vi "Random Seas (math only).vi"() -> ()   [LabVIEW 2012]
uses:
  Instance           2 19Saved   Random Seas .vi
  Instance           1 19Saved   Random Seas .vi
panel:
  out "File Name Out":path
  out "Wavestaff Signal":dbl[](graph)
  in  "Measure Waves":bool
  in  "Input Settings":bool
  in  "Geometric Settings":bool
  in  "Limit Settings":bool
  in  "Output Settings":bool
  out "Output Sig. Wave Height":dbl format="%.4f"
  out "Buffer Completed":dbl format="%.1f"
  out "Time Series Data":dbl[](array[numeric]) format="%.2f"
  out "Output Signal":dbl[](graph)
  in  "Set spectal parameters":bool
  in  "Run":bool
  in  "Power":bool
  out "Significant Wave Period":dbl format="%.4f"
  out "Significant Wave Height":dbl format="%.4f"
  in  "Select spectrum":u16(ring) items=["Bretschnieder", "JONSWAP", "NH Extreme", "NH Typical", "Pierson Moskowitz"]
  out "Spectra":cluster{"Numeric":dbl, "Numeric":dbl}[](graph)
  out "Time Series":cluster{"Numeric":dbl, "Numeric":sgl}[](graph)
  # "Random Sea Generator"
  # "m"
  # "s"
  # "Time (min:sec)"
  # "%"
  # "m"
  # "Time (min:sec)"
  # "Frequency (Hz)"
  # "Advanced"
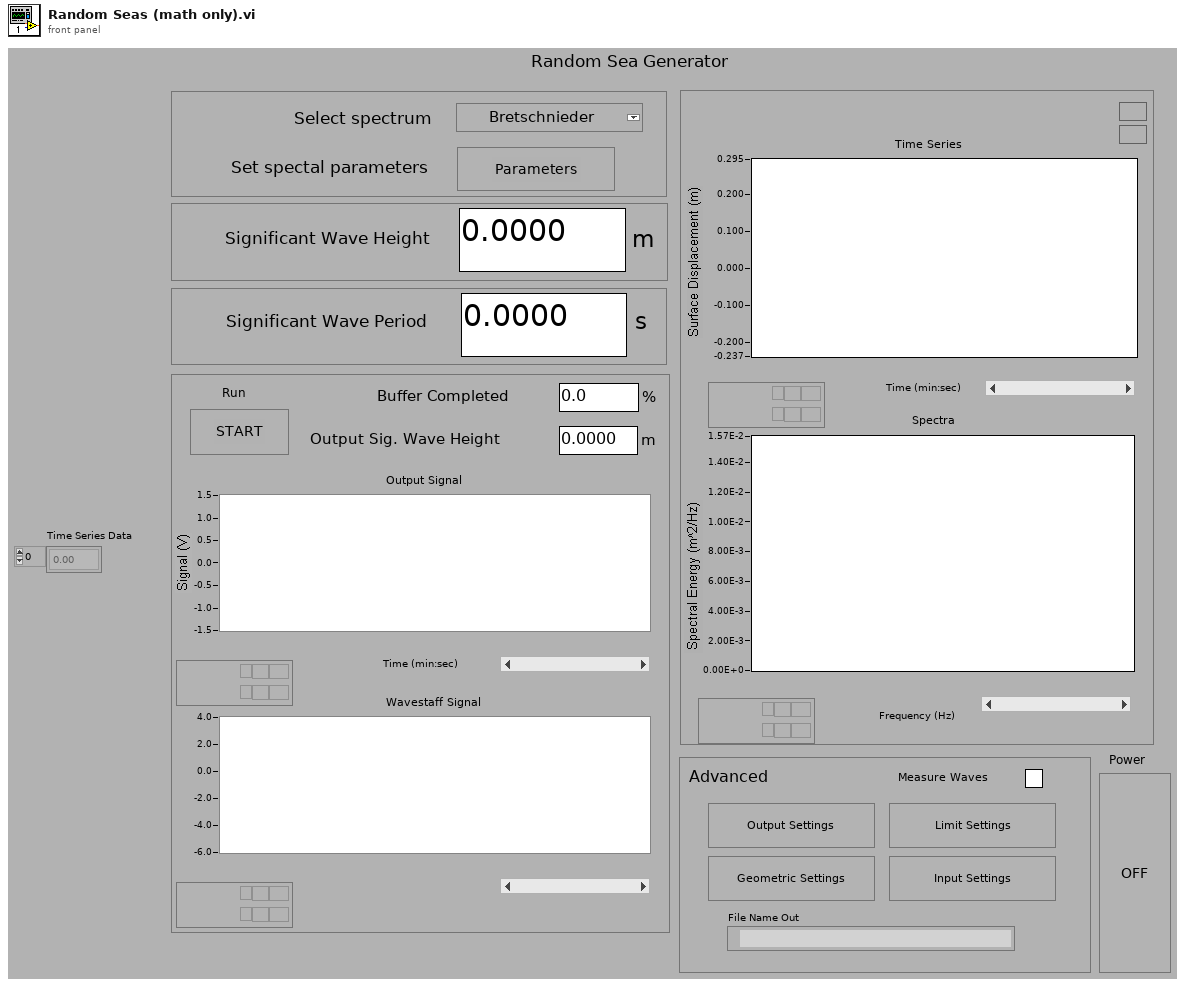
[diagram p1: front panel]
types:
  T1 = cluster{"Input Device":i32, "Input Channel":string, "Input Offset":dbl, "Input Calibration":dbl}
  T2 = cluster{"Device":i16, "Channel":string, "Sampling Rate":i32, "Ramp Time":dbl, "Buffer Length":u16, "Buffer Size":i32, "Sub Buffer Length":i16, "Sub Buffer Size":i16}
  T3 = cluster{"Stroke Calibration":dbl, "Water Depth":dbl, "Paddle Height":dbl}
  T4 = cluster{"Min Wave Period":dbl, "Max Wave Period":dbl, "Cutoff Frequency":dbl, "Max 1/2 Piston Stroke":dbl, "Max H/L":dbl, "Max H/d":dbl}
  T5 = cluster{"Bretschneider":cluster{"Sig Wave Height":dbl, "Sig Wave Period":dbl, "Scale Ratio":dbl}, "JONSWAP":cluster{"Sig Wave Height":dbl, "Sig Wave Period":dbl, "Gamma":dbl, "Sigma A":dbl, "Sigma B":dbl, "Scale Ratio":dbl}, "NH Extreme":cluster{"Sig Wave Height":dbl, "Sig Wave Period":dbl, "Gamma":dbl, "Sigma A":dbl, "Sigma B":dbl, "P":dbl, "Scale Ratio":dbl}, "NH Typical":cluster{"Sig Wave Height":dbl, "Sig Wave Period 1":dbl, "Sig Wave Period 2":dbl, "Gamma 1":dbl, "Gamma 2":dbl, "P":dbl, "Scale Ratio":dbl}, "PM":cluster{"Wind speed":dbl, "Scale Ratio":dbl}}
  T6 = cluster{"Element Data":dbl, "Element Data":dbl}[]
  T7 = cluster{"Sig Wave Height":dbl, "Sig Wave Period":dbl, "Scale Ratio":dbl}
  T8 = cluster{"Sig Wave Height":dbl, "Sig Wave Period":dbl, "Gamma":dbl, "Sigma A":dbl, "Sigma B":dbl, "Scale Ratio":dbl}
  T9 = cluster{"Sig Wave Height":dbl, "Sig Wave Period":dbl, "Gamma":dbl, "Sigma A":dbl, "Sigma B":dbl, "P":dbl, "Scale Ratio":dbl}
  T10 = cluster{"Sig Wave Height":dbl, "Sig Wave Period":dbl, "Sig Wave Period 2":dbl, "Gamma 1":dbl, "Gamma 2":dbl, "P":dbl, "Scale Ratio":dbl}
  T11 = cluster{"Device":i16, "Channel":string, "Sampling Rate":i32, "Stroke Calibration":dbl, "Buffer Length":u16, "Buffer Size":i32, "Sub Buffer Length":i16, "Sub Buffer Size":i16}
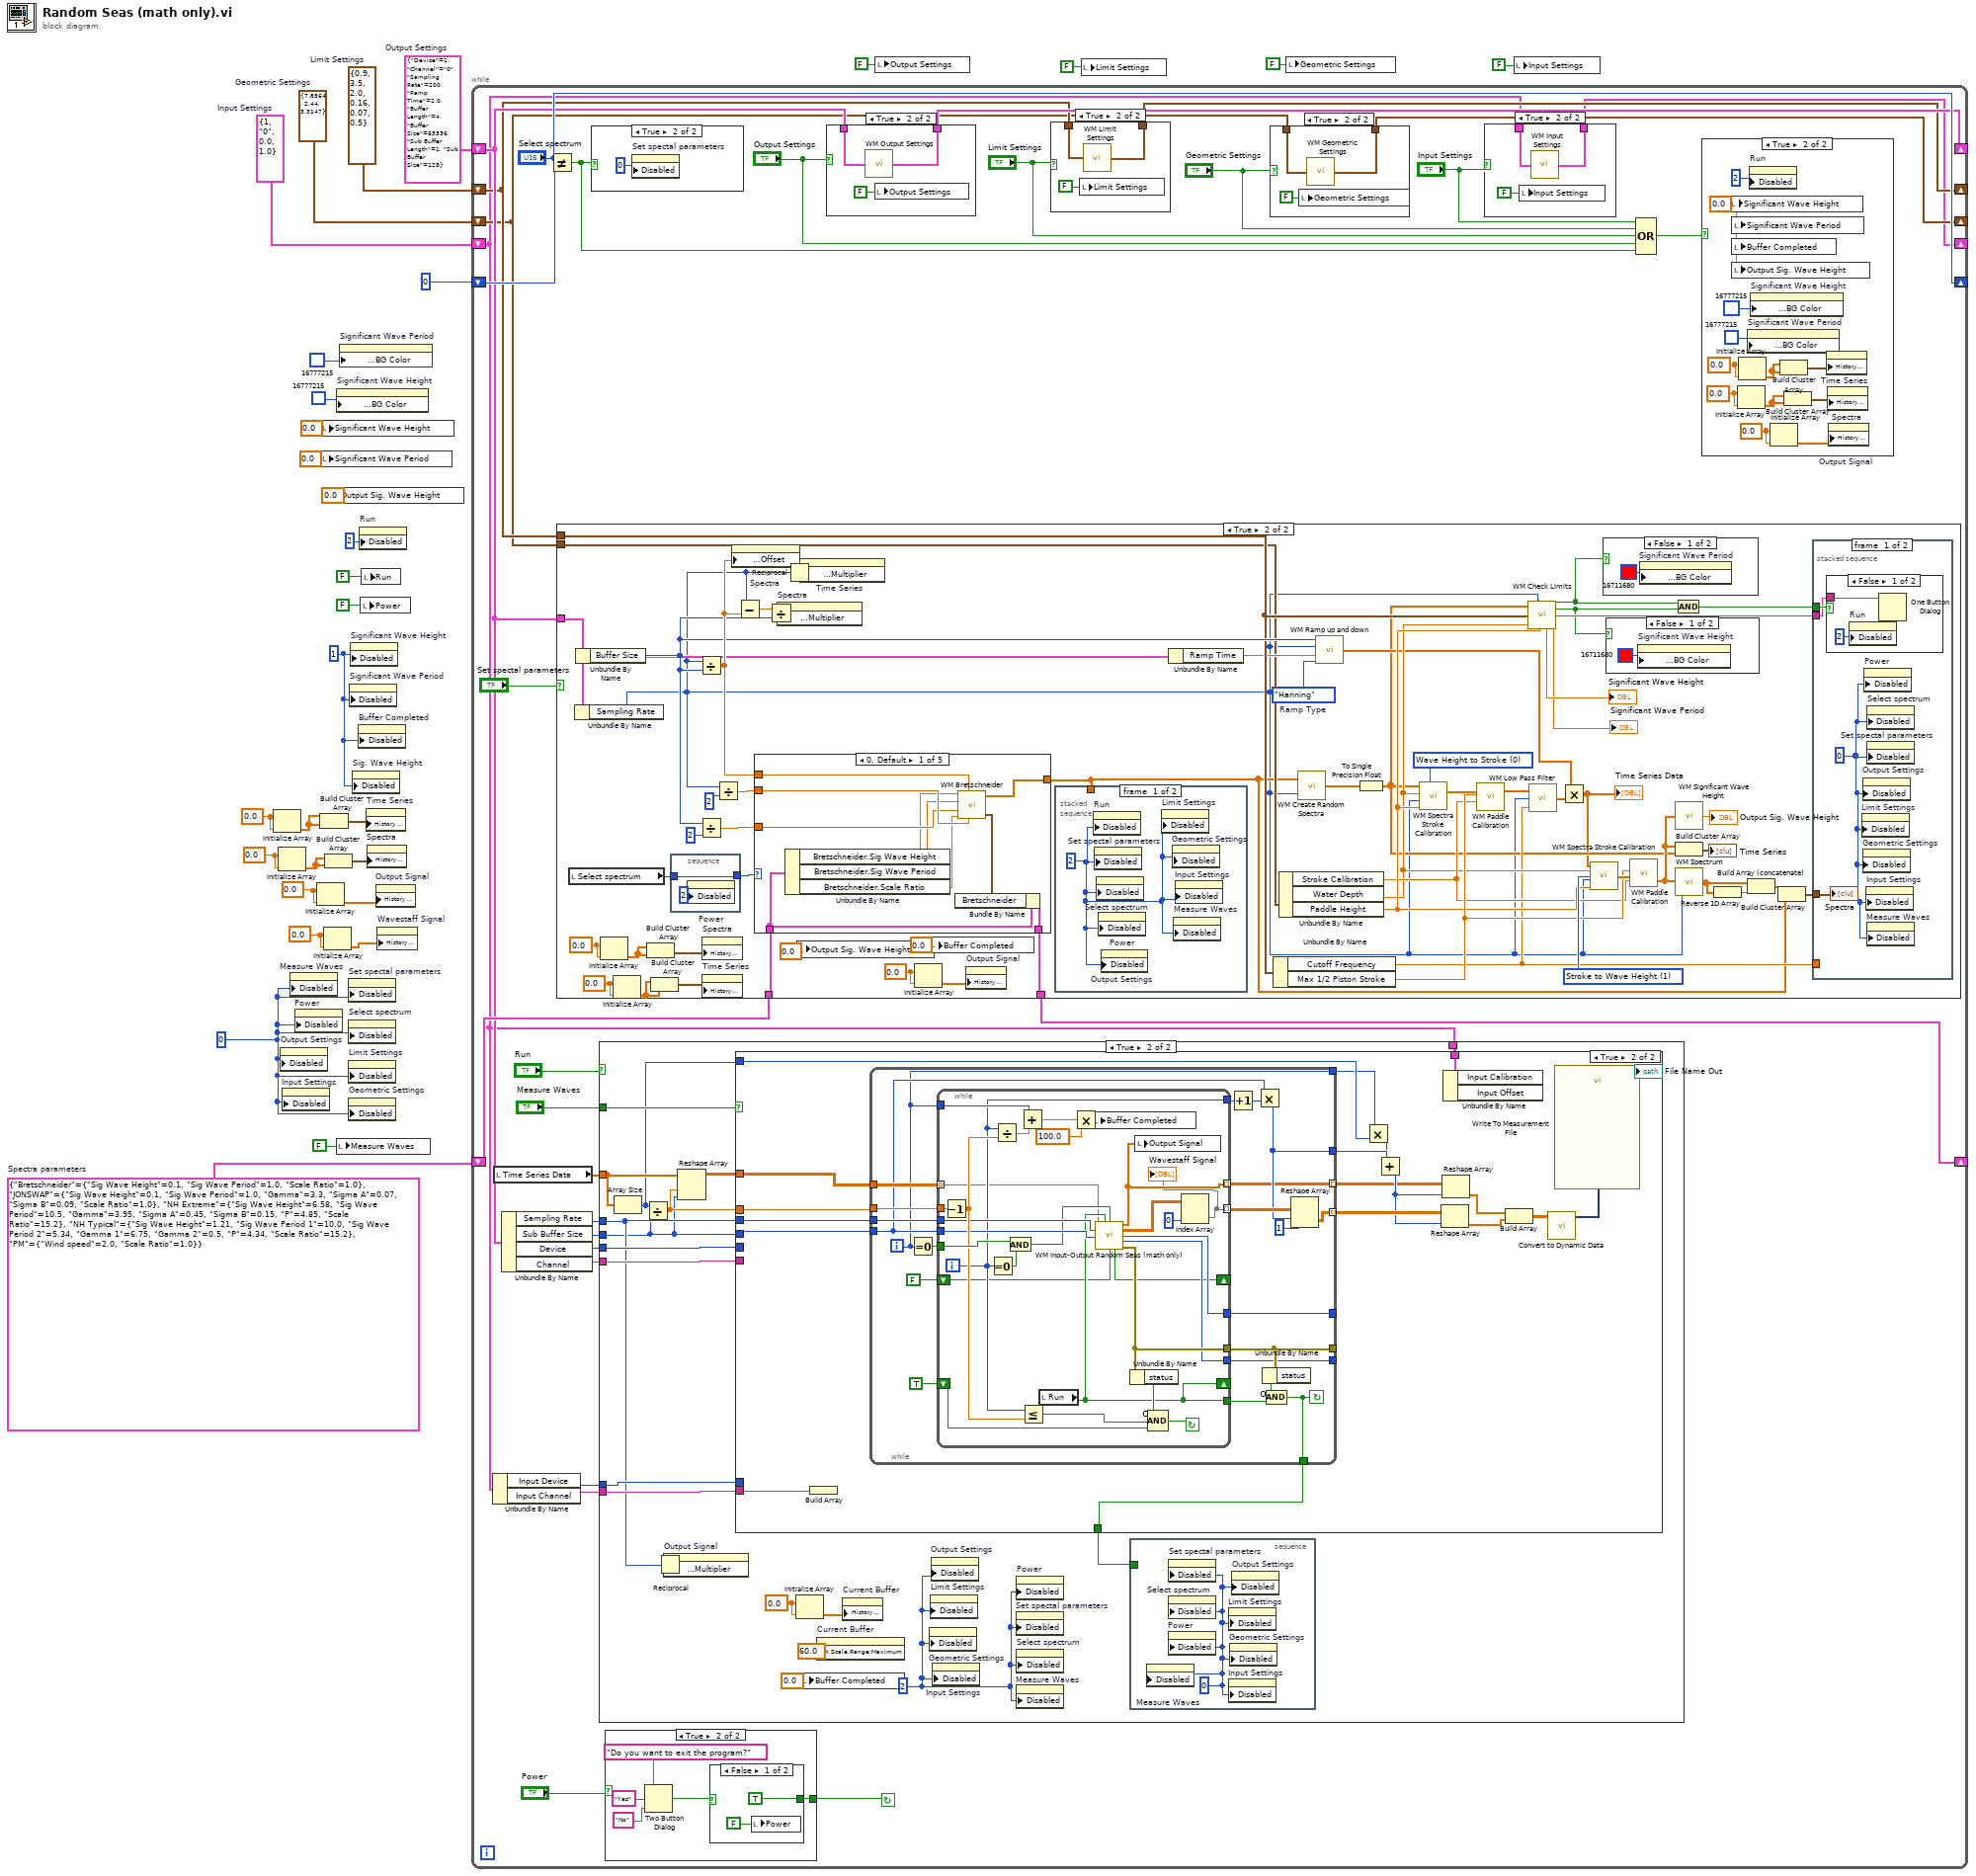
[diagram p0: block diagram]
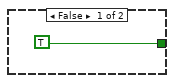
[diagram p7: hidden frame]
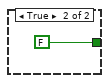
[diagram p8: hidden frame]
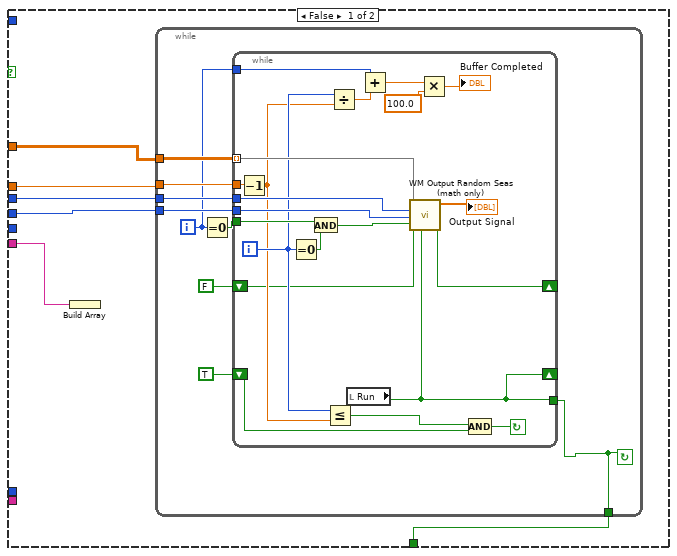
[diagram p11: hidden frame]
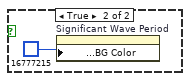
[diagram p13: hidden frame]
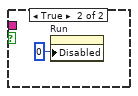
[diagram p15: hidden frame]
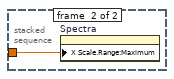
[diagram p16: hidden frame]
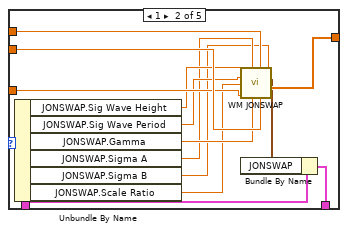
[diagram p17: hidden frame]
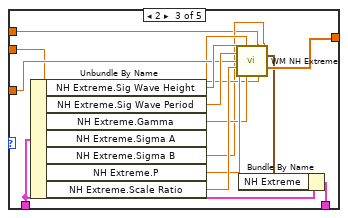
[diagram p18: hidden frame]
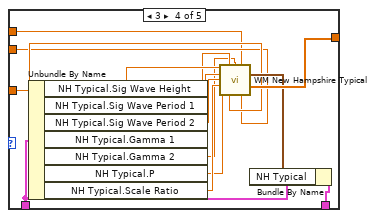
[diagram p19: hidden frame]
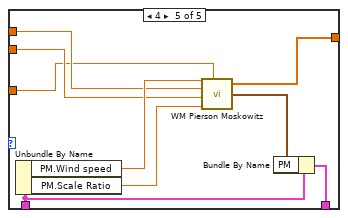
[diagram p20: hidden frame]
diagram:
  w2 = 0.0 ("Element Data")
  w5 = T1 {"Input Device"=1, "Input Channel"="0", "Input Offset"=0.0, "Input Calibration"=1.0}  # Input Settings
  w8 = T2 {"Device"=1, "Channel"="0", "Sampling Rate"=200, "Ramp Time"=2.0, "Buffer Length"=4, "Buffer Size"=65536, "Sub Buffer Length"=1, "Sub Buffer Size"=128}  # Output Settings
  w10 = T3 {"Stroke Calibration"=7.8564, "Water Depth"=2.44, "Paddle Height"=3.3147}  # Geometric Settings
  w11 = T4 {"Min Wave Period"=0.9, "Max Wave Period"=3.5, "Cutoff Frequency"=2.0, "Max 1/2 Piston Stroke"=0.16, "Max H/L"=0.07, "Max H/d"=0.5}  # Limit Settings
  w16 = 0.0 ("Element Data")
  w3 = u8 0 ("Write Attribute")
  w27 = 0.0 ("Element Data")
  w28 = 0.0 ("Element Data")
  w25 = T5 {"Bretschneider"={"Sig Wave Height"=0.1, "Sig Wave Period"=1.0, "Scale Ratio"=1.0}, "JONSWAP"={"Sig Wave Height"=0.1, "Sig Wave Period"=1.0, "Gamma"=3.3, "Sigma A"=0.07, "Sigma B"=0.09, "Scale Ratio"=1.0}, "NH Extreme"={"Sig Wave Height"=6.58, "Sig Wave Period"=10.5, "Gamma"=3.95, "Sigma A"=0.45, "Sigma B"=0.15, "P"=4.85, "Scale Ratio"=15.2}, "NH Typical"={"Sig Wave Height"=1.21, "Sig Wave Period 1"=10.0, "Sig Wave Period 2"=5.34, "Gamma 1"=6.75, "Gamma 2"=0.5, "P"=4.34, "Scale Ratio"=15.2}, "PM"={"Wind speed"=2.0, "Scale Ratio"=1.0}}  # Spectra parameters
  w9 = 1
  n1 = Initialize Array(w28, w28) -> (w18:dbl[])
  n2 = Initialize Array(w27, w27) -> (w26:dbl[])
  n3 = property on="Output Settings" class="Bool (strict)"("Disabled"=w3) -> ()  [unwired: 2 in, 2 out]
  n4 = property on="Input Settings" class="Bool (strict)"("Disabled"=w3) -> ()  [unwired: 2 in, 2 out]
  n5 = property on="Measure Waves" class="Bool (strict)"("Disabled"=w3) -> ()  [unwired: 2 in, 2 out]
  n6 = property on="Power" class="Bool (strict)"("Disabled"=w3) -> ()  [unwired: 2 in, 2 out]
  n7 = Initialize Array(w16, w16) -> (w15:dbl[])
  n8 = local write "Significant Wave Height"(0.0 ("Significant Wave Height")) -> ()
  n9 = local write "Significant Wave Period"(0.0 ("Significant Wave Period")) -> ()
  n10 = Build Cluster Array(w18, w18) -> (w17:T6)
  n11 = Initialize Array(w2, w2) -> (w1:dbl[])
  n12 = Build Cluster Array(w26, w26) -> (w19:T6)
  n13 = local write "Output Sig. Wave Height"(0.0 ("Sig. Wave Height")) -> ()
  n14 = property on="Significant Wave Height" class="DigNum (strict)"("Numeric Text.Text Colors:BG Color"=u32 16777215) -> ()  [unwired: 2 in, 2 out]
  n15 = local write "Measure Waves"(FALSE ("Measure Waves")) -> ()
  n16 = property on="Significant Wave Period" class="DigNum (strict)"("Numeric Text.Text Colors:BG Color"=u32 16777215) -> ()  [unwired: 2 in, 2 out]
  n17 = property on="Set spectal parameters" class="Bool"("Disabled"=w3) -> ()  [unwired: 2 in, 2 out]
  n18 = property on="Select spectrum" class="Ring (strict)"("Disabled"=w3) -> ()  [unwired: 2 in, 2 out]
  n19 = property on="Limit Settings" class="Bool (strict)"("Disabled"=w3) -> ()  [unwired: 2 in, 2 out]
  n20 = property on="Geometric Settings" class="Bool (strict)"("Disabled"=w3) -> ()  [unwired: 2 in, 2 out]
  n21 = property on="Significant Wave Period" class="DigNum (strict)"("Disabled"=w9) -> ()  [unwired: 2 in, 2 out]
  n22 = property on="Significant Wave Height" class="DigNum (strict)"("Disabled"=w9) -> ()  [unwired: 2 in, 2 out]
  n23 = property on="Sig. Wave Height" class="DigNum (strict)"("Disabled"=w9) -> ()  [unwired: 2 in, 2 out]
  n24 = property on="Buffer Completed" class="DigNum (strict)"("Disabled"=w9) -> ()  [unwired: 2 in, 2 out]
  n25 = property on="Run" class="Bool (strict)"("Disabled"=u8 2 ("Write Attribute")) -> ()  [unwired: 2 in, 2 out]
  n26 = local write "Power"(FALSE ("Power")) -> ()
  n27 = local write "Run"(FALSE ("Run")) -> ()
  n28 = property on="Time Series" class="WFChart (strict)"("History Data"=w17) -> ()  [unwired: 2 in, 2 out]
  n29 = property on="Spectra" class="WFChart (strict)"("History Data"=w19) -> ()  [unwired: 2 in, 2 out]
  n30 = property on="Output Signal" class="WFChart (strict)"("History Data"=w15) -> ()  [unwired: 2 in, 2 out]
  n31 = property on="Wavestaff Signal" class="WFChart (strict)"("History Data"=w1) -> ()  [unwired: 2 in, 2 out]
  n32 = while {
    shift-left: w5 -> [w32]
    shift-right: [w42] -> _
    shift-left: w10 -> [w43]
    shift-right: [w44] -> _
    shift-left: w11 -> [w45]
    shift-right: [w46] -> _
    shift-left: w8 -> [w51]
    shift-right: [w52] -> _
    shift-left: 0 -> [w55]
    shift-right: ["Select spectrum"] -> _
    shift-left: w25 -> [w60]
    shift-right: [w59] -> _
    stop <- w54 continue-if-true
    n33 = Unbundle By Name(w32) -> ("Input Device"=w34:i32, "Input Channel"=w33:string)
    n34 = local read "Time Series Data"() -> (w58:dbl[])
    n35 = Unbundle By Name(w51) -> ("Sampling Rate"=w50:i32, "Sub Buffer Size"=w49:i16, "Device"=w48:i16, "Channel"=w47:string)
    n36 = Not Equal?(x="Select spectrum", y=w55) -> (x != y?=w41:bool)
    n37 = case shown="True" "Set spectal parameters" {
      tunnel: [w224 w248] -> w59
      tunnel: w60 -> [w224 w272]
      tunnel: w51 -> [_ w235]
      tunnel: w45 -> [_ w239]
      tunnel: w43 -> [_ w237]
      frame False {
      }
      frame True {
        w246 = u16 0 items=["Wave Height to Stroke", "Stroke to Wave Height"] ("Conversion Type")
        w247 = u16 1 items=["Wave Height to Stroke", "Stroke to Wave Height"] ("Conversion Type")
        w271 = enum16{"Linear", "Hanning"}."Hanning"  # Ramp Type
        w257 = 0.0 ("Element Data")
        w269 = 0.0 ("Element Data")
        w279 = 0.0 ("Element Data")
        n38 = local read "Select spectrum"() -> (w259:u16)
        n39 = Unbundle By Name(w235) -> ("Sampling Rate"=w225:i32)
        n40 = Unbundle By Name(w235) -> ("Buffer Size"=w249:i32)
        n41 = Initialize Array(w269, w269) -> (w268:dbl[])
        n42 = Initialize Array(w279, w279) -> (w266:dbl[])
        n43 = Build Cluster Array(w268, w268) -> (w267:T6)
        n44 = Build Cluster Array(w266, w266) -> (w265:T6)
        n45 = stacked-sequence {
          tunnel: w259 -> [w286]
          tunnel: [w286] -> w258
          frame #0 {
            n46 = property on="Power" class="Bool (strict)"("Disabled"=u8 2 ("Write Attribute")) -> ()  [unwired: 2 in, 2 out]
          }
        }
        n47 = Divide(x=w225, y=w249) -> (x/y=w276:dbl)
        n48 = Divide(x=w249, y=2) -> (x/y=w278:dbl)
        n49 = property on="Spectra" class="WFChart (strict)"("History Data"=w267) -> ()  [unwired: 2 in, 2 out]
        n50 = property on="Time Series" class="WFChart (strict)"("History Data"=w265) -> ()  [unwired: 2 in, 2 out]
        n51 = Divide(x=w225, y=i8 2) -> (x/y=w277:dbl)
        n52 = property on="Spectra" class="WFChart (strict)"("X Scale.Offset and Multiplier:Offset"=w276) -> ()  [unwired: 2 in, 2 out]
        n53 = Subtract(x=w225, y=w276) -> (x-y=w280:dbl)
        n54 = case shown="0, Default" w258 {
          tunnel: [w305 w315 w322 w346 w352] -> w227
          tunnel: w278 -> [w302 w316 w330 w335 w347]
          tunnel: w277 -> [w303 w317 w326 w334 w348]
          tunnel: w276 -> [w304 w318 w323 w333 w349]
          tunnel: [w298 w306 w320 w345 w354] -> w248
          tunnel: w272 -> [w300 w308 w321 w343 w355]
          frame 0, Default {
            n55 = Unbundle By Name(w300) -> ("Bretschneider.Sig Wave Height"=w297:dbl, "Bretschneider.Sig Wave Period"=w296:dbl, "Bretschneider.Scale Ratio"=w301:dbl)
            n56 = call "WM Bretschneider.vi"("Significant Wave Height"=w297, "Start Freq"=w304, "Peak Wave Period"=w296, "Number of Frequencies"=w302, "End Freq"=w303, "Scale Ratio"=w301) -> ("Spectral Energy"=w305:dbl[], "Bretschneider parameters"=w299:T7)  [unwired: 1 out]
            n57 = Bundle By Name(cluster=w300, "Bretschneider"=w299) -> (w298:T5)
          }
          frame 1 {
            n58 = Unbundle By Name(w308) -> ("JONSWAP.Sig Wave Height"=w314:dbl, "JONSWAP.Sig Wave Period"=w313:dbl, "JONSWAP.Gamma"=w312:dbl, "JONSWAP.Sigma A"=w311:dbl, "JONSWAP.Sigma B"=w310:dbl, "JONSWAP.Scale Ratio"=w309:dbl)
            n59 = call "WM JONSWAP.vi"("Sigma B"=w310, "End Freq (Model Scale)"=w317, "Start Freq (Model Scale)"=w318, "Gamma"=w312, "Sigma A"=w311, "Number of Frequencies"=w316, "Scale Ratio"=w309, "Peak Wave Period"=w313, "Significant Wave Height"=w314) -> ("Spectral Energy"=w315:dbl[], "JONSWAP parameters"=w307:T8)  [unwired: 1 out]
            n60 = Bundle By Name(cluster=w308, "JONSWAP"=w307) -> (w306:T5)
          }
          frame 2 {
            n61 = Unbundle By Name(w321) -> ("NH Extreme.Sig Wave Height"=w332:dbl, "NH Extreme.Sig Wave Period"=w331:dbl, "NH Extreme.Gamma"=w327:dbl, "NH Extreme.Sigma A"=w325:dbl, "NH Extreme.Sigma B"=w324:dbl, "NH Extreme.P"=w328:dbl, "NH Extreme.Scale Ratio"=w329:dbl)
            n62 = call "WM NH Extreme.vi"("Significant Wave Height"=w332, "Sigma A"=w325, "Start Freq (Model Scale)"=w323, "Sigma B"=w324, "Peak Wave Period"=w331, "Number of Frequencies"=w330, "Scale Ratio"=w329, "P"=w328, "Gamma"=w327, "End Freq (Model Scale)"=w326) -> ("NH Extreme parameters"=w319:T9, "Spectral Energy"=w322:dbl[])  [unwired: 3 in, 1 out]
            n63 = Bundle By Name(cluster=w321, "NH Extreme"=w319) -> (w320:T5)
          }
          frame 3 {
            n64 = Unbundle By Name(w343) -> ("NH Typical.Sig Wave Height"=w342:dbl, "NH Typical.Sig Wave Period 1"=w341:dbl, "NH Typical.Sig Wave Period 2"=w340:dbl, "NH Typical.Gamma 1"=w337:dbl, "NH Typical.Gamma 2"=w336:dbl, "NH Typical.P"=w338:dbl, "NH Typical.Scale Ratio"=w339:dbl)
            n65 = call "WM New Hampshire Typical.vi"("Significant Wave Height"=w342, "Gamma 1"=w337, "Gamma 2"=w336, "Start Freq (Model Scale)"=w333, "Peak Wave Period 1"=w341, "Peak Wave Period 2"=w340, "Scale Ratio"=w339, "P"=w338, "Number of Frequencies"=w335, "End Freq (Model Scale)"=w334) -> ("NH Typical parameters"=w344:T10, "Spectral Energy"=w346:dbl[])  [unwired: 3 in, 1 out]
            n66 = Bundle By Name(cluster=w343, "NH Typical"=w344) -> (w345:T5)
          }
          frame 4 {
            n67 = Unbundle By Name(w355) -> ("PM.Wind speed"=w351:dbl, "PM.Scale Ratio"=w350:dbl)
            n68 = call "WM Pierson Moskowitz.vi"("Wind Speed"=w351, "Start Freq (Model Scale)"=w349, "End Freq (Model Scale)"=w348, "Scale Ratio"=w350, "Number of Frequencies"=w347) -> ("Spectral Energy"=w352:dbl[], "PM parameters"=w353:cluster{"Wind Speed":dbl, "Scale Ratio":dbl})  [unwired: 1 out]
            n69 = Bundle By Name(cluster=w355, "PM"=w353) -> (w354:T5)
          }
        }
        n70 = Divide(x=w280, y=w249) -> (x/y=w275:dbl)
        n71 = property on="Spectra" class="WFChart (strict)"("X Scale.Offset and Multiplier:Multiplier"=w275) -> ()  [unwired: 2 in, 2 out]
        n72 = Reciprocal(x=w225) -> (1/x=w254:dbl)
        n73 = local write "Output Sig. Wave Height"(0.0 ("Sig. Wave Height")) -> ()
        n74 = property on="Time Series" class="WFChart (strict)"("X Scale.Offset and Multiplier:Multiplier"=w254) -> ()  [unwired: 2 in, 2 out]
        n75 = Initialize Array(w257, w257) -> (w256:dbl[])
        n76 = local write "Buffer Completed"(0.0 ("Buffer Completed")) -> ()
        n77 = property on="Output Signal" class="WFChart (strict)"("History Data"=w256) -> ()  [unwired: 2 in, 2 out]
        n78 = stacked-sequence {
          tunnel: w227 -> [_ _]
          frame #0 {
            w287 = u8 2 ("Write Attribute")
            n79 = property on="Run" class="Bool (strict)"("Disabled"=w287) -> ()  [unwired: 2 in, 2 out]
            n80 = property on="Set spectal parameters" class="Bool"("Disabled"=w287) -> ()  [unwired: 2 in, 2 out]
            n81 = property on="Select spectrum" class="Ring (strict)"("Disabled"=w287) -> ()  [unwired: 2 in, 2 out]
            n82 = property on="Power" class="Bool (strict)"("Disabled"=w287) -> ()  [unwired: 2 in, 2 out]
            n83 = property on="Output Settings" class="Bool (strict)"("Disabled"=w287) -> ()  [unwired: 2 in, 2 out]
            n84 = property on="Limit Settings" class="Bool (strict)"("Disabled"=w287) -> ()  [unwired: 2 in, 2 out]
            n85 = property on="Geometric Settings" class="Bool (strict)"("Disabled"=w287) -> ()  [unwired: 2 in, 2 out]
            n86 = property on="Measure Waves" class="Bool (strict)"("Disabled"=w287) -> ()  [unwired: 2 in, 2 out]
            n87 = property on="Input Settings" class="Bool (strict)"("Disabled"=w287) -> ()  [unwired: 2 in, 2 out]
          }
          frame #1 {
          }
        }
        n88 = Unbundle By Name(w235) -> ("Ramp Time"=w238:dbl)
        n89 = Unbundle By Name(w239) -> ("Cutoff Frequency"=w231:dbl, "Max 1/2 Piston Stroke"=w240:dbl)
        n90 = Unbundle By Name(w237) -> ("Stroke Calibration"=w234:dbl, "Water Depth"=w233:dbl, "Paddle Height"=w236:dbl)
        n91 = call "WM Create Random Spectra.vi"("Sampling Freq"=w225, "Wave Spectra"=w227) -> ("Time Series"=w230:dbl[])
        n92 = call "WM Ramp up and down.vi"("Ramp Type"=w271, "Ramp Time"=w238, "Sampling Rate"=w225, "Buffer Size"=w249) -> ("Output"=w229:dbl[])
        n93 = To Single Precision Float(number=w230) -> (single precision float=w228:sgl[])
        n94 = call "WM Spectra Stroke Calibration.vi"("Input Time Series"=w228, "Water Depth"=w233, "Sampling Rate"=w225, "Paddle Height"=w236, "Conversion Type"=w246) -> ("Output Time Series"=w264:dbl[])
        n95 = call "WM Paddle Calibration.vi"("Stroke Calibration (V/m)"=w234, "Max 1/2 Piston Stroke (m)"=w240, "Input Stroke Distance (m)"=w264) -> ("Output Voltage"=w263:dbl[])  [unwired: 1 in, 1 out]
        n96 = call "WM Check Limits.vi"("Input Time Series"=w228, "Sampling Rate (Hz)"=w225, "Limit Settings"=w239, "Water Depth (m)"=w233, "Paddle Height (m)"=w236) -> ("Wave Period OK"=w242:bool, "Wave Height OK"=w243:bool, "Error Message"=w253:string, "Significant Wave Height (m)"=→"Significant Wave Height":dbl, "Significant Wave Period (s)"=→"Significant Wave Period":dbl)
        n97 = call "WM Low Pass Filter.vi"("Cutoff Freq"=w231, "Sampling Freq"=w225, "Input"=w263) -> ("Output"=w261:dbl[])
        n98 = Multiply(x=w229, y=w261) -> (x*y=w226:dbl[])
        "Time Series Data" <- w226
        n99 = call "WM Spectra Stroke Calibration.vi"("Input Time Series"=w226, "Water Depth"=w233, "Sampling Rate"=w225, "Paddle Height"=w236, "Conversion Type"=w247) -> ("Output Time Series"=w241:dbl[])
        n100 = case shown="False" w242 {
          frame False {
            n101 = property on="Significant Wave Period" class="DigNum (strict)"("Numeric Text.Text Colors:BG Color"=u32 16711680) -> ()  [unwired: 2 in, 2 out]
          }
          frame True {
            n102 = property on="Significant Wave Period" class="DigNum (strict)"("Numeric Text.Text Colors:BG Color"=u32 16777215) -> ()  [unwired: 2 in, 2 out]
          }
        }
        n103 = case shown="False" w243 {
          frame False {
            n104 = property on="Significant Wave Height" class="DigNum (strict)"("Numeric Text.Text Colors:BG Color"=u32 16711680) -> ()  [unwired: 2 in, 2 out]
          }
          frame True {
            n105 = property on="Significant Wave Height" class="DigNum (strict)"("Numeric Text.Text Colors:BG Color"=u32 16777215) -> ()  [unwired: 2 in, 2 out]
          }
        }
        n106 = call "WM Paddle Calibration.vi"("Input Voltage"=w241, "Stroke Calibration (V/m)"=w234, "Max 1/2 Piston Stroke (m)"=w240) -> ("Output Stroke Distance"=w252:dbl[])  [unwired: 1 in, 1 out]
        n107 = And(x=w242, y=w243) -> (x .and. y?=w260:bool)
        n108 = Build Cluster Array(w252, w228) -> (→"Time Series":cluster{"Numeric":dbl, "Numeric":sgl}[])
        n109 = call "WM Spectrum.vi"("Sampling Rate"=w225, "Time Series"=w252) -> ("Spectra"=w274:dbl[])
        n110 = call "WM Significant Wave Height.vi"("Input"=w252) -> ("Significant Wave Height"=→"Output Sig. Wave Height":dbl)
        n111 = Reverse 1D Array(array=w274) -> (reversed array=w273:dbl[])
        n112 = Build Array (concatenate)(w274, w273) -> (w270:dbl[])
        n113 = Build Cluster Array(w270, w227) -> (w232:cluster{"Numeric":dbl, dbl}[])
        n114 = stacked-sequence {
          tunnel: w232 -> [w291 _]
          tunnel: w260 -> [w290 _]
          tunnel: w253 -> [w289 _]
          tunnel: w231 -> [_ w295]
          frame #0 {
            w288 = u8 0 ("Write Attribute")
            n115 = case shown="False" w290 {
              tunnel: w289 -> [w292 _]
              frame False {
                n116 = property on="Run" class="Bool (strict)"("Disabled"=u8 2 ("Write Attribute")) -> ()  [unwired: 2 in, 2 out]
                n117 = One Button Dialog(message=w292) -> ()  [unwired: 1 in, 1 out]
              }
              frame True {
                n118 = property on="Run" class="Bool (strict)"("Disabled"=u8 0 ("Write Attribute")) -> ()  [unwired: 2 in, 2 out]
              }
            }
            n119 = property on="Limit Settings" class="Bool (strict)"("Disabled"=w288) -> ()  [unwired: 2 in, 2 out]
            n120 = property on="Output Settings" class="Bool (strict)"("Disabled"=w288) -> ()  [unwired: 2 in, 2 out]
            n121 = property on="Geometric Settings" class="Bool (strict)"("Disabled"=w288) -> ()  [unwired: 2 in, 2 out]
            n122 = property on="Power" class="Bool (strict)"("Disabled"=w288) -> ()  [unwired: 2 in, 2 out]
            n123 = property on="Input Settings" class="Bool (strict)"("Disabled"=w288) -> ()  [unwired: 2 in, 2 out]
            n124 = property on="Select spectrum" class="Ring (strict)"("Disabled"=w288) -> ()  [unwired: 2 in, 2 out]
            n125 = property on="Set spectal parameters" class="Bool"("Disabled"=w288) -> ()  [unwired: 2 in, 2 out]
            n126 = property on="Measure Waves" class="Bool (strict)"("Disabled"=w288) -> ()  [unwired: 2 in, 2 out]
            "Spectra" <- w291
          }
          frame #1 {
            n127 = property on="Spectra" class="WFChart (strict)"("X Scale.Range:Maximum"=w295) -> ()  [unwired: 2 in, 2 out]
          }
        }
      }
    }
    n128 = case shown="True" w41 {
      frame False {
      }
      frame True {
        n129 = property on="Set spectal parameters" class="Bool"("Disabled"=u8 0 ("Write Attribute")) -> ()  [unwired: 2 in, 2 out]
      }
    }
    n130 = case shown="True" "Run" {
      tunnel: w58 -> [_ w106]
      tunnel: w50 -> [_ w107]
      tunnel: w49 -> [_ w103]
      tunnel: w48 -> [_ w114]
      tunnel: w47 -> [_ w113]
      tunnel: "Measure Waves" -> [_ w112]
      tunnel: w34 -> [_ w111]
      tunnel: w33 -> [_ w110]
      tunnel: w32 -> [_ w102]
      frame False {
      }
      frame True {
        w101 = u8 2 ("Write Attribute")
        w118 = 0.0 ("Element Data")
        n131 = Array Size(array=w106) -> (size(s)=w100:i32)
        n132 = Divide(x=w100, y=w103) -> (x/y=w104:dbl)
        n133 = Reciprocal(x=w107) -> (1/x=w108:dbl)
        n134 = property on="Output Signal" class="WFChart (strict)"("X Scale.Offset and Multiplier:Multiplier"=w108) -> ()  [unwired: 2 in, 2 out]
        n135 = Reshape Array(w106, w104, w103) -> (w105:dbl[][])
        n136 = case shown="True" w112 {
          tunnel: w105 -> [w121 w171]
          tunnel: w107 -> [w124 w172]
          tunnel: w103 -> [w123 w167]
          tunnel: w114 -> [_ _]
          tunnel: w113 -> [w122 _]
          tunnel: w111 -> [_ _]
          tunnel: w110 -> [_ w173]
          tunnel: [w119 w169] -> w109
          tunnel: w104 -> [w120 w170]
          tunnel: w102 -> [_ w168]
          tunnel: w100 -> [_ w163]
          frame False {
            n137 = Build Array(w122) -> ()  [unwired: 1 out]
            n138 = while {
              tunnel: w124 -> [w130]
              tunnel: [w125] -> w119
              tunnel: w120 -> [w131]
              tunnel: w123 -> [w133]
              tunnel: w121 -> [w132]
              i -> [w128]
              stop <- w125 continue-if-true
              n139 = Equal To 0?(x=w128) -> (x = 0?=w129:bool)
              n140 = while {
                shift-left: TRUE ("Run") -> [w134]
                shift-right: [w135] -> _
                shift-left: FALSE ("End Out") -> [w136]
                shift-right: [w137] -> _
                tunnel: w128 -> [w144]
                tunnel: w130 -> [w150]
                tunnel: [w135] -> w125
                tunnel: w131 -> [w152]
                tunnel: w132 -> [w145] mode=indexing
                tunnel: w129 -> [w153]
                tunnel: w133 -> [w151]
                i -> [w143]
                stop <- w149 continue-if-true
                n141 = Decrement(x=w152) -> (x-1=w141:dbl)
                n142 = Equal To 0?(x=w143) -> (x = 0?=w154:bool)
                n143 = And(x=w153, y=w154) -> (x .and. y?=w148:bool)
                n144 = Less Or Equal?(x=w143, y=w141) -> (x <= y?=w146:bool)
                n145 = Divide(x=w143, y=w141) -> (x/y=w142:dbl)
                n146 = local read "Run"() -> (w135:bool)
                n147 = Add(x=w144, y=w142) -> (x+y=w140:dbl)
                n148 = call "WM Output Random Seas (math only).vi"("Start up"=w148, "Run"=w135, "End"=w136, "Sub Buffer Size"=w151, "Sampling Rate"=w150, "Input Time Series"=w145) -> ("End Out"=w137:bool, "Buffer"=→"Output Signal":dbl[])  [unwired: 4 in]
                n149 = Multiply(x=w140, y=100.0) -> (x*y=→"Buffer Completed":dbl)
                n150 = Compound Arithmetic op=AND(w146, w134) -> (w149:bool)
              }
            }
          }
          frame True {
            n151 = Build Array(w173) -> ()  [unwired: 1 out]
            n152 = while {
              tunnel: [w176] -> w166
              tunnel: [w179] -> w162
              tunnel: [w177] -> w165 mode=indexing
              tunnel: [w184] -> _
              tunnel: [w188] -> _
              tunnel: [w187] -> _
              tunnel: w172 -> [w189]
              tunnel: [w190] -> w169
              tunnel: w170 -> [w192]
              tunnel: w167 -> [w181]
              tunnel: w171 -> [w194]
              tunnel: [w174] -> w159 mode=indexing
              i -> [w179]
              stop <- w190 continue-if-true
              n153 = Equal To 0?(x=w179) -> (x = 0?=w186:bool)
              n154 = while {
                shift-left: FALSE ("End Out") -> [w198]
                shift-right: [w199] -> _
                tunnel: [w201] -> w183
                tunnel: [w195] -> w178 mode=indexing
                tunnel: [w204] -> w184
                tunnel: w179 -> [w215]
                tunnel: [w206] -> w188
                tunnel: [w205] -> w187
                tunnel: w189 -> [w210]
                tunnel: [w208] -> w191
                tunnel: w192 -> [w219]
                shift-left: TRUE ("StartStop") -> [w220]
                shift-right: [w208] -> _
                tunnel: w194 -> [w197] mode=indexing
                tunnel: w186 -> [w221]
                tunnel: w181 -> [w209]
                tunnel: [w196] -> w174 mode=indexing
                i -> [w201]
                stop <- w218 continue-if-true
                n155 = Decrement(x=w219) -> (x-1=w213:dbl)
                n156 = Equal To 0?(x=w201) -> (x = 0?=w222:bool)
                n157 = Divide(x=w201, y=w213) -> (x/y=w214:dbl)
                n158 = And(x=w221, y=w222) -> (x .and. y?=w207:bool)
                n159 = Add(x=w215, y=w214) -> (x+y=w212:dbl)
                n160 = Less Or Equal?(x=w201, y=w213) -> (x <= y?=w216:bool)
                n161 = local read "Run"() -> (w208:bool)
                n162 = Multiply(x=w212, y=100.0) -> (x*y=w203:dbl)
                n163 = local write "Buffer Completed"(w203) -> ()
                n164 = call "WM Input-Output Random Seas (math only).vi"("Output Time Series"=w197, "Run"=w208, "Start up/Continue"=w207, "Sampling Rate"=w210, "Sub Buffer Size"=w209, "End"=w198) -> ("Buffer"=w196:dbl[], "Experimental Data"=w200:dbl[][], "Output Task ID Out"=w206:u32, "Input Task ID Out"=w204:u32, "End Out"=w199:bool, "error out"=w205:errorcluster)  [unwired: 4 in]
                n165 = Unbundle By Name(w205) -> ("status"=w217:bool)
                n166 = local write "Output Signal"(w196) -> ()
                n167 = Compound Arithmetic op=AND(invert w217, w216, w220) -> (w218:bool)
                n168 = Index Array(array=w200, index (col)=0 ("Index")) -> (element=w195:dbl[])  [unwired: 1 in]
                "Wavestaff Signal" <- w195
              }
              n169 = Increment(x=w183) -> (x+1=w182:i32)
              n170 = Multiply(x=w181, y=w182) -> (x*y=w176:i32)
              n171 = Unbundle By Name(w187) -> ("status"=w185:bool)
              n172 = Compound Arithmetic op=AND(invert w185, w191) -> (w190:bool)
              n173 = Reshape Array(w178, w176, 1 ("Dimension Size")) -> (w177:dbl[][])
            }
            n174 = Multiply(x=w162, y=w163) -> (x*y=w164:i32)
            n175 = Add(x=w164, y=w166) -> (x+y=w160:i32)
            n176 = Reshape Array(w165, w160) -> (w161:dbl[])
            n177 = Reshape Array(w159, w160) -> (w158:dbl[])
            n178 = Unbundle By Name(w168) -> ()  [unwired: 2 out]
            n179 = Build Array(w158, w161) -> (w157:dbl[][])
            n180 = call "Convert to Dynamic Data"("2D Array"=w157) -> ("Dynamic Data Type"=w156:dynamicdata)  [unwired: 3 in]
            n181 = call "Write To Measurement File"("Signals"=w156) -> ("File Name Out"=→"File Name Out":path)  [unwired: 16 in, 2 out]
          }
        }
        n182 = Initialize Array(w118, w118) -> (w117:dbl[])
        n183 = local write "Buffer Completed"(0.0 ("Buffer Completed")) -> ()
        n184 = property on="Current Buffer" class="WFChart (strict)"("X Scale.Range:Maximum"=60.0 ("Write Attribute")) -> ()  [unwired: 2 in, 2 out]
        n185 = property on="Current Buffer" class="WFChart (strict)"("History Data"=w117) -> ()  [unwired: 2 in, 2 out]
        n186 = property on="Geometric Settings" class="Bool (strict)"("Disabled"=w101) -> ()  [unwired: 2 in, 2 out]
        n187 = property on="Limit Settings" class="Bool (strict)"("Disabled"=w101) -> ()  [unwired: 2 in, 2 out]
        n188 = property on="Output Settings" class="Bool (strict)"("Disabled"=w101) -> ()  [unwired: 2 in, 2 out]
        n189 = property on="Input Settings" class="Bool (strict)"("Disabled"=w101) -> ()  [unwired: 2 in, 2 out]
        n190 = property on="Power" class="Bool (strict)"("Disabled"=w101) -> ()  [unwired: 2 in, 2 out]
        n191 = property on="Set spectal parameters" class="Bool"("Disabled"=w101) -> ()  [unwired: 2 in, 2 out]
        n192 = property on="Select spectrum" class="Ring (strict)"("Disabled"=w101) -> ()  [unwired: 2 in, 2 out]
        n193 = property on="Measure Waves" class="Bool (strict)"("Disabled"=w101) -> ()  [unwired: 2 in, 2 out]
        n194 = stacked-sequence {
          tunnel: w109 -> [_]
          frame #0 {
            w223 = 0
            n195 = property on="Measure Waves" class="Bool (strict)"("Disabled"=w223) -> ()  [unwired: 2 in, 2 out]
            n196 = property on="Set spectal parameters" class="Bool"("Disabled"=w223) -> ()  [unwired: 2 in, 2 out]
            n197 = property on="Select spectrum" class="Ring (strict)"("Disabled"=w223) -> ()  [unwired: 2 in, 2 out]
            n198 = property on="Power" class="Bool (strict)"("Disabled"=w223) -> ()  [unwired: 2 in, 2 out]
            n199 = property on="Limit Settings" class="Bool (strict)"("Disabled"=w223) -> ()  [unwired: 2 in, 2 out]
            n200 = property on="Input Settings" class="Bool (strict)"("Disabled"=w223) -> ()  [unwired: 2 in, 2 out]
            n201 = property on="Geometric Settings" class="Bool (strict)"("Disabled"=w223) -> ()  [unwired: 2 in, 2 out]
            n202 = property on="Output Settings" class="Bool (strict)"("Disabled"=w223) -> ()  [unwired: 2 in, 2 out]
          }
        }
      }
    }
    n203 = case shown="True" "Power" {
      tunnel: [TRUE w91] -> w54
      frame False {
      }
      frame True {
        n204 = Two Button Dialog(message="Do you want to exit the program?", 1:"No" ("F button name (\"Cancel\")"), 2:"Yes" ("T button name (\"OK\")")) -> (T button?=w92:bool)
        n205 = case shown="False" w92 {
          tunnel: [TRUE FALSE] -> w91
          frame False {
            n206 = local write "Power"(FALSE ("Power")) -> ()
          }
          frame True {
          }
        }
      }
    }
    n207 = case shown="True" "Output Settings" {
      tunnel: w51 -> [w86 w87]
      tunnel: [w86 w89] -> w52
      frame False {
      }
      frame True {
        n208 = call "WM Output Settings.vi"("Output Settings"=w87) -> ("Output Settings Results"=w89:T11)
        n209 = local write "Output Settings"(FALSE ("Output Settings")) -> ()
      }
    }
    n210 = case shown="True" "Limit Settings" {
      tunnel: w45 -> [w82 w84]
      tunnel: [w82 w83] -> w46
      frame False {
      }
      frame True {
        n211 = local write "Limit Settings"(FALSE ("Limit Settings")) -> ()
        n212 = call "WM Limit Settings.vi"("Limit Settings"=w84) -> ("Limit Settings Output"=w83:T4)
      }
    }
    n213 = case shown="True" "Geometric Settings" {
      tunnel: w43 -> [w78 w81]
      tunnel: [w78 w80] -> w44
      frame False {
      }
      frame True {
        n214 = local write "Geometric Settings"(FALSE ("Geometric Settings")) -> ()
        n215 = call "WM Geometric Settings.vi"("Geometric Settings"=w81) -> ("Geometric Settings Output"=w80:T3)
      }
    }
    n216 = case shown="True" "Input Settings" {
      tunnel: w32 -> [w74 w75]
      tunnel: [w74 w76] -> w42
      frame False {
      }
      frame True {
        n217 = local write "Input Settings"(FALSE ("Input Settings")) -> ()
        n218 = call "WM Input Settings.vi"("Input Settings"=w75) -> ("Input Settings Out"=w76:T1)
      }
    }
    n219 = Compound Arithmetic op=OR("Input Settings", "Geometric Settings", "Limit Settings", "Output Settings", w41) -> (w36:bool)
    n220 = case shown="True" w36 {
      frame False {
      }
      frame True {
        w63 = 0.0 ("Element Data")
        w68 = 0.0 ("Element Data")
        w69 = 0.0 ("Element Data")
        w72 = 0.0 ("Significant Wave Height")
        n221 = local write "Significant Wave Height"(w72) -> ()
        n222 = local write "Significant Wave Period"(w72) -> ()
        n223 = local write "Buffer Completed"(w72) -> ()
        n224 = local write "Output Sig. Wave Height"(w72) -> ()
        n225 = Initialize Array(w68, w68) -> (w67:dbl[])
        n226 = Initialize Array(w69, w69) -> (w65:dbl[])
        n227 = property on="Significant Wave Period" class="DigNum (strict)"("Numeric Text.Text Colors:BG Color"=u32 16777215) -> ()  [unwired: 2 in, 2 out]
        n228 = property on="Run" class="Bool (strict)"("Disabled"=u8 2 ("Write Attribute")) -> ()  [unwired: 2 in, 2 out]
        n229 = property on="Significant Wave Height" class="DigNum (strict)"("Numeric Text.Text Colors:BG Color"=u32 16777215) -> ()  [unwired: 2 in, 2 out]
        n230 = Initialize Array(w63, w63) -> (w62:dbl[])
        n231 = Build Cluster Array(w65, w65) -> (w64:T6)
        n232 = Build Cluster Array(w67, w67) -> (w66:T6)
        n233 = property on="Time Series" class="WFChart (strict)"("History Data"=w64) -> ()  [unwired: 2 in, 2 out]
        n234 = property on="Spectra" class="WFChart (strict)"("History Data"=w66) -> ()  [unwired: 2 in, 2 out]
        n235 = property on="Output Signal" class="WFChart (strict)"("History Data"=w62) -> ()  [unwired: 2 in, 2 out]
      }
    }
  }
  n236 = local write "Output Settings"(FALSE ("Output Settings")) -> ()
  n237 = local write "Limit Settings"(FALSE ("Limit Settings")) -> ()
  n238 = local write "Geometric Settings"(FALSE ("Geometric Settings")) -> ()
  n239 = local write "Input Settings"(FALSE ("Input Settings")) -> ()
